vi "Spreadsheet Storage(OpenWriteClose).vi"() -> ()   [LabVIEW 2017]
panel:
  in  "Waveform Parameters":T1={"Frequency"=50.0, "Amplitude"=5.0, "Shape"=enum."Sine"}
  in  "Digitizing Parameters":T2={"Numbers of Samples"=10, "Sampling Frequency"=1000.0}
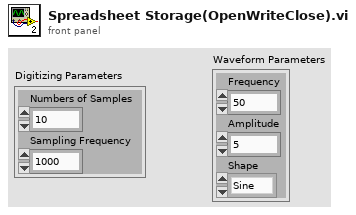
[diagram p1: front panel]
types:
  T1 = cluster{"Frequency":dbl, "Amplitude":dbl, "Shape":enum16{"Sine", "Cosine", "DC Level", "Square", "User-Defined"}}
  T2 = cluster{"Numbers of Samples":i32, "Sampling Frequency":dbl}
  T3 = enum16{"open", "replace", "create", "open or create", "replace or create", "replace or create with confirmation"}
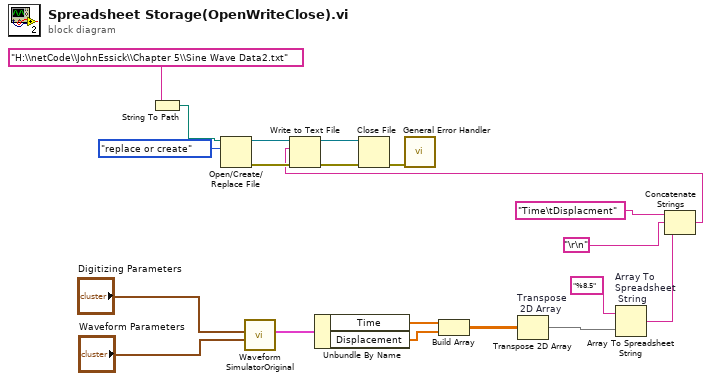
[diagram p0: block diagram]
diagram:
  n1 = String To Path(string="H:\\netCode\\JohnEssick\\Chapter 5\\Sine Wave Data2.txt" ("format (%.3f)")) -> (path=w15:path)
  n2 = Open/Create/Replace File(file path (use dialog)=w15, operation (0:open)=T3."replace or create") -> (refnum out=w14:refnum<file>, error out=w12:errorcluster)  [unwired: 4 in, 1 out]
  n3 = call "Waveform SimulatorOriginal.vi"("Waveform Parameters"="Waveform Parameters", "Digitizing Parameters"="Digitizing Parameters") -> ("Waveform Output"=w18:cluster{"Time":dbl[], "Displacement":dbl[]})  [unwired: 9 in]
  n4 = Unbundle By Name "Unbundle By Name"(w18) -> ("Time"=w17:dbl[], "Displacement"=w16:dbl[])
  n5 = Build Array "Build Array"(w17, w16) -> (w8:dbl[][])
  n6 = Transpose 2D Array "Transpose\n 2D Array"(2D array=w8) -> (transposed array=w7:dbl[][])
  n7 = Array To Spreadsheet String "Array To \nSpreadsheet\n String"(array=w7, 3:"%8.5" ("format string")) -> (spreadsheet string=w2:string)  [unwired: 1 in]
  n8 = Concatenate Strings("Time\tDisplacment", "\r\n", w2) -> (w1:string)
  n9 = Write to Text File(file (use dialog)=w14, text=w1, error in=w12) -> (refnum out=w13:refnum<file>, error out=w11:errorcluster)  [unwired: 1 in, 1 out]
  n10 = Close File(refnum=w13, error in=w11) -> (error out=w10:errorcluster)  [unwired: 1 out]
  n11 = call <vilib>:"General Error Handler.vi"("error in (no error)"=w10) -> ()  [unwired: 10 in, 5 out]
